vi "MeasureExportStrings.vi"() -> ()   [LabVIEW 2012]
panel:
  out "MeasureExportStrings":string[](array[string])
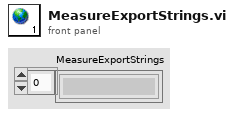
[diagram p1: front panel]
diagram:
